vi "InitiateStriptest.vi"   [LabVIEW 2013]
doc: "General utility to start striptests with a probe card."
uses:
  InstrControl/InstrumentSetup.vi
  InstrControl/InstrControl.lvclass
  InstrControl/ProbeStationControl/ProbeStationControl.lvclass
types:
  T1 = enum16{"Striptest", "IV & CV", "Interstrip Cap", "Interstrip Res", "Current Stability", "IV Loop"}
  T2 = enum16{"Striptest", "IV", "CV", "Interstrip Cap", "Interstrip Res", "Stability", "Test", "Nothing"}
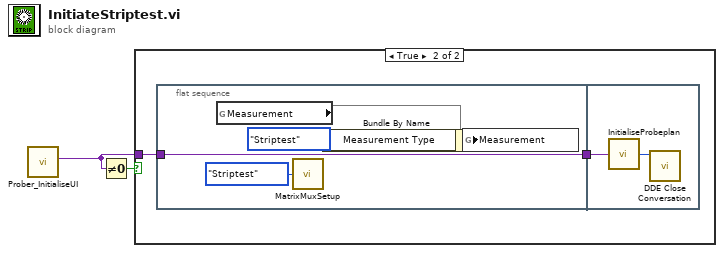
[diagram p0: block diagram]
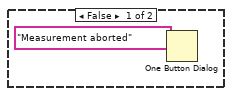
[diagram p2: hidden frame]
diagram:
  n1 = call-dynamic "Prober_InitialiseUI.vi"() -> ("Probestation Configuration"=w1:variant)  [unwired: 9 in, 2 out]
  n2 = Not Equal To 0?(x=w1) -> (x != 0?=w2:bool)
  n3 = case shown="True" w2 {
    tunnel: w1 -> [_ w5]
    frame False {
      n4 = One Button Dialog(message="Measurement aborted") -> ()  [unwired: 1 in, 1 out]
    }
    frame True {
      n5 = flat-sequence {
        tunnel: w5 -> [w10]
        tunnel: [w10] -> w4
        tunnel: w4 -> [w12]
        frame #0 {
          n6 = global read "InstrumentSetup.vi" "Measurement"() -> (w9)
          n7 = call "MatrixMuxSetup.vi"("Measurement"=T2."Striptest") -> ()
          n8 = Bundle By Name(cluster=w9, "Measurement Type"=T1."Striptest") -> (w8:cluster{})
          n9 = global write "InstrumentSetup.vi" "Measurement"(w8) -> ()
        }
        frame #1 {
          n10 = call "InitialiseProbeplan.vi"("Ref No. In"=w12) -> ("Ref No. Out"=w11:u32)
          n11 = call <vilib>:"DDE Close Conversation.vi"("conversation refnum"=w11) -> ()  [unwired: 8 in, 1 out]
        }
      }
    }
  }
